vi "Write Output_Enable.vi"(8 "error in":errorcluster, 10 "Output_Enable":bool, 11 "PowerSupply in":refnum<class "PowerSupply.lvclass">) -> (0 "error out":errorcluster, 3 "PowerSupply out":refnum<class "PowerSupply.lvclass">)   [LabVIEW 2019, in "PowerSupply.lvlib" / "PowerSupply.lvclass"]
uses:
  Library/PowerSupply.lvclass
  C:/Users/Public/Documents/Development/builds/Engine/Monitored Actor.lvlibp/Monitored Actor/Monitored Actor/Monitored Actor.lvclass
  Library/PowerSupply.lvclass/PowerSupply.ctl
  Read Settings.vi
  Write Settings.vi
  Private/Accessors/Read Is UUT Supply.vi
  builds/Engine/Monitored Actor.lvlibp/Monitored Actor/Monitored Actor/Read Actor Label.vi
  builds/Engine/Engine.lvlibp/Project/Engine.lvclass
  builds/Instruments/Instruments.lvlibp/Library/Instruments.lvclass
  builds/Instruments/Instruments.lvlibp/Private/Polymorphic/Special/Event from Boolean.vi
  builds/Instruments/Instruments.lvlibp
  C:/Users/Public/Documents/Development/builds/Instruments/Instruments.lvlibp/Library/Instruments.lvclass
  C:/Users/Public/Documents/Development/builds/Tools/Config.lvlibp/Config.lvclass
  C:/Users/Public/Documents/Development/builds/Engine/Engine.lvlibp/Project/Engine.lvclass
  C:/Users/Public/Documents/Development/builds/Engine/Panel Manager.lvlibp/Panel Actor/Panel Actor.lvclass
  C:/Users/Public/Documents/Development/builds/Engine/Actor Framework.lvlibp/1abvi3w/vi.lib/ActorFramework/Actor/Actor.lvclass
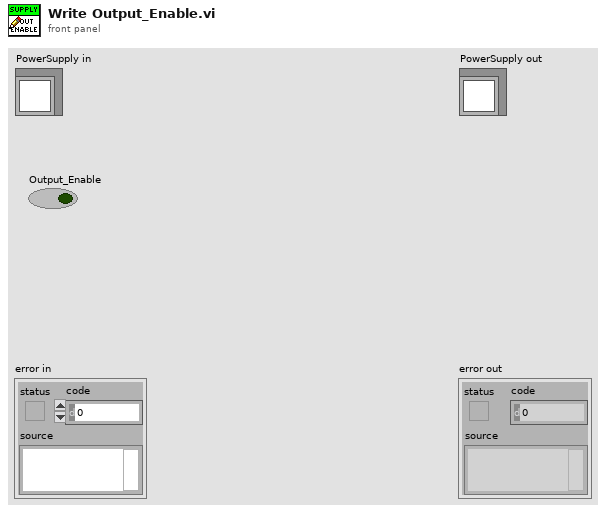
[diagram p1: front panel]
types:
  T1 = typedef "PowerSupply.lvlib/PowerSupply.lvclass/Settings.ctl" = cluster{"Voltage":dbl, "Current":dbl, "Output":bool, "OverVolt_Protect":dbl, "OverCurrent_Protect":dbl, "OVP":bool, "OCP":bool, "Interlock":bool, "Volt_Ramp":dbl, "Current_Ramp":dbl, "Sense Point":T2, "OCP Mode":T3}
  T2 = typedef "PowerSupply.lvlib/PowerSupply.lvclass/Sense Point.ctl" = enum16{"Local", "Remote"}
  T3 = typedef "PowerSupply.lvlib/PowerSupply.lvclass/OCP Mode.ctl" = enum16{"Shutdown", "Foldback"}
  T4 = cluster{"Timestamp":timestamp, "Description":string, "Data":string}
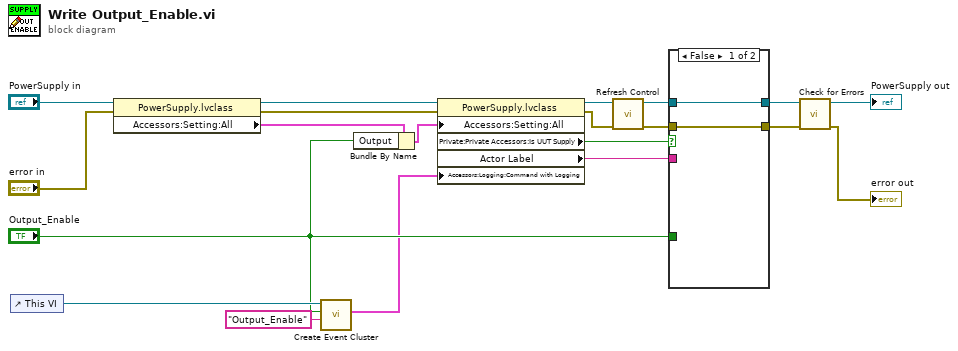
[diagram p0: block diagram]
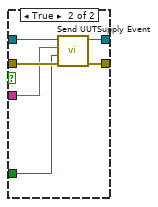
[diagram p2: hidden frame]
diagram:
  n1 = control-ref of="This VI"() -> (w4:refnum<vi>)
  n2 = property class="PowerSupply.lvclass"(reference="PowerSupply in", error in="error in") -> (reference out=w20:refnum<class "PowerSupply.lvclass">, error out=w12:errorcluster, "Accessors:Setting:All"=w14:T1)
  n3 = call-poly "Create Event Cluster.vi"("Name"="Output_Enable", "Value"="Output_Enable", "VI Refnum"=w4) -> ("Event Data"=w1:T4)  [unwired: 8 in]
  n4 = Bundle By Name(cluster=w14, "Output"="Output_Enable") -> (w13:T1)
  n5 = property class="PowerSupply.lvclass"(reference=w20, error in=w12, "Accessors:Setting:All"=w13, "Accessors:Logging:Command with Logging"=w1) -> (reference out=w19:refnum<class "PowerSupply.lvclass">, error out=w11:errorcluster, "Private:Private Accessors:Is UUT Supply"=w6:bool, "Actor Label"=w5:string)
  n6 = call "Refresh Control.vi"("error in"=w11, "PowerSupply in"=w19) -> ("error out"=w9:errorcluster, "PowerSupply out"=w10:refnum<class "PowerSupply.lvclass">)  [unwired: 8 in]
  n7 = case shown="False" w6 {
    tunnel: w10 -> [w22 w28]
    tunnel: w9 -> [w21 w27]
    tunnel: [w22 w26] -> w8
    tunnel: [w21 w25] -> w7
    tunnel: w5 -> [_ w24]
    tunnel: "Output_Enable" -> [_ w23]
    frame False {
    }
    frame True {
      n8 = call "Send UUTSupply Event.vi"("error in"=w27, "Output"=w23, "Supply"=w24, "Engine in"=w28) -> ("error out"=w25:errorcluster, "Engine out"=w26:refnum<class "PowerSupply.lvclass">)  [unwired: 6 in]
    }
  }
  n9 = call "Check for Errors.vi"("error in"=w7, "Engine in"=w8) -> ("error out"=→"error out":errorcluster, "Engine out"=→"PowerSupply out":refnum<class "PowerSupply.lvclass">)  [unwired: 8 in]
